vi "Recognize Starting Point.vi"() -> (0 "Sorted Waypoints":T1[](array[typedef]) {"Longitude" format="%#_14g"; "Latitude" format="%#_14g"}, 3 "Starting WP":T1={"Latitude"=2560.754484, "Longitude"=4991.702604} {"Longitude" format="%#_14g"; "Latitude" format="%#_14g"})   [LabVIEW 2009]
uses:
  TypeDefs/Sensor Typedefs/GPS Data.ctl
panel:
  out "Starting Point Index":i32=1
  out "Distances":dbl[](array[numeric])=[34.68592578168008, 0.0, 17.48374136365253]
  in  "NDIA GPS Pt":T1={"Latitude"=2560.745094, "Longitude"=4991.701278} {"Longitude" format="%#_14g"; "Latitude" format="%#_14g"}
  in  "SAIC GPS Pt":T1={"Latitude"=2560.754484, "Longitude"=4991.702604} {"Longitude" format="%#_14g"; "Latitude" format="%#_14g"}
  in  "Oakland GPS Pt":T1={"Latitude"=2560.7532, "Longitude"=4991.72802} {"Longitude" format="%#_14g"; "Latitude" format="%#_14g"}
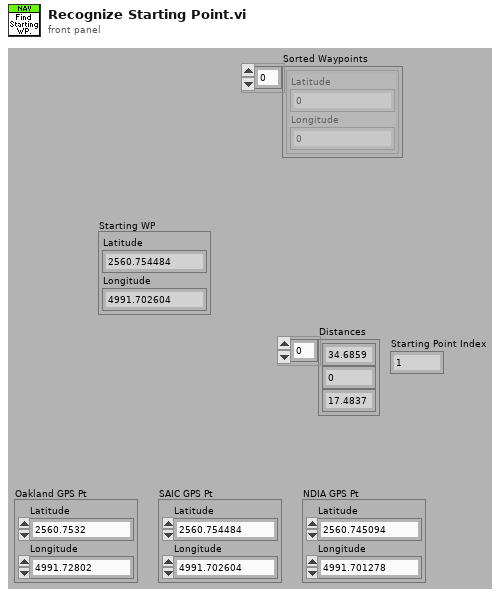
[diagram p1: front panel]
types:
  T1 = typedef "GPS Data.ctl" = cluster{"Latitude":dbl, "Longitude":dbl}
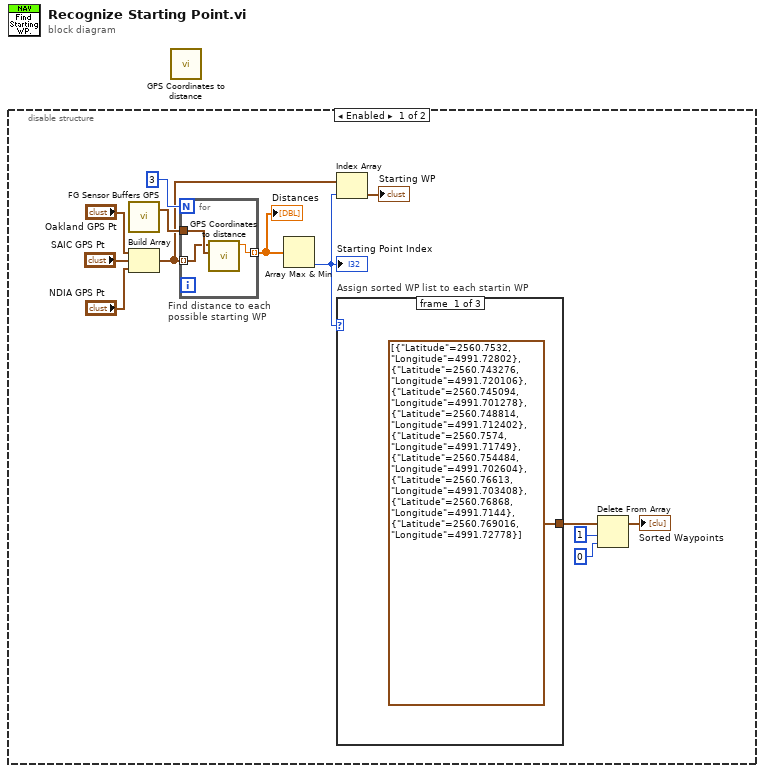
[diagram p0: block diagram]
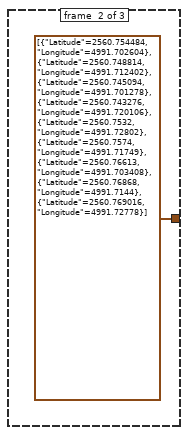
[diagram p2: hidden frame]
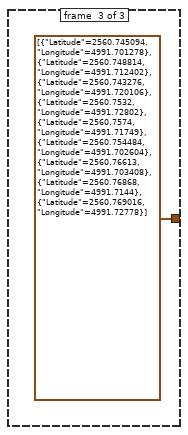
[diagram p3: hidden frame]
diagram:
  n1 = disable-structure shown="Enabled" {
    frame #0 {
      n2 = call "FG Sensor Buffers GPS.vi"() -> ("GPS Buffer out"=w13:T1)  [unwired: 3 in]
      n3 = Build Array("Oakland GPS Pt", "SAIC GPS Pt", "NDIA GPS Pt") -> (w7:T1[])
      n4 = for "Find distance to each\npossible starting WP" {
        N: 3 -> [_]
        tunnel: w13 -> [w19]
        tunnel: w7 -> [w18] mode=indexing
        tunnel: [w17] -> w8 mode=indexing
        n5 = call "GPS Coordinates to distance.vi"("GPS Co-ordinate 2"=w19, "GPS Co-ordinate 1"=w18) -> ("Distance"=w17:dbl)  [unwired: 9 in]
      }
      "Distances" <- w8
      n6 = Array Max & Min(array=w8) -> (min index (indices)=w5:i32)  [unwired: 3 out]
      "Starting Point Index" <- w5
      n7 = Index Array(array=w7, index=w5) -> (element=→"Starting WP":T1)
      n8 = case "Assign sorted WP list to each startin WP" shown="2" w5 {
        tunnel: [T1[] [{"Latitude"=2560.7532, "Longitude"=4991.72802}, {"Latitude"=2560.743276, "Longitude"=4991.720106}, {"Latitude"=2560.745094, "Longitude"=4991.701278}, {"Latitude"=2560.748814, "Longitude"=4991.712402}, {"Latitude"=2560.7574, "Longitude"=4991.71749}, {"Latitude"=2560.754484, "Longitude"=4991.702604}, {"Latitude"=2560.76613, "Longitude"=4991.703408}, {"Latitude"=2560.76868, "Longitude"=4991.7144}, {"Latitude"=2560.769016, "Longitude"=4991.72778}] T1[] [{"Latitude"=2560.754484, "Longitude"=4991.702604}, {"Latitude"=2560.748814, "Longitude"=4991.712402}, {"Latitude"=2560.745094, "Longitude"=4991.701278}, {"Latitude"=2560.743276, "Longitude"=4991.720106}, {"Latitude"=2560.7532, "Longitude"=4991.72802}, {"Latitude"=2560.7574, "Longitude"=4991.71749}, {"Latitude"=2560.76613, "Longitude"=4991.703408}, {"Latitude"=2560.76868, "Longitude"=4991.7144}, {"Latitude"=2560.769016, "Longitude"=4991.72778}] T1[] [{"Latitude"=2560.745094, "Longitude"=4991.701278}, {"Latitude"=2560.748814, "Longitude"=4991.712402}, {"Latitude"=2560.743276, "Longitude"=4991.720106}, {"Latitude"=2560.7532, "Longitude"=4991.72802}, {"Latitude"=2560.7574, "Longitude"=4991.71749}, {"Latitude"=2560.754484, "Longitude"=4991.702604}, {"Latitude"=2560.76613, "Longitude"=4991.703408}, {"Latitude"=2560.76868, "Longitude"=4991.7144}, {"Latitude"=2560.769016, "Longitude"=4991.72778}]] -> w4
        frame #0 {
        }
        frame #1 {
        }
        frame #2 {
        }
      }
      n9 = Delete From Array(array=w4, length=1, index=0) -> (array with subset deleted=→"Sorted Waypoints":T1[])  [unwired: 1 out]
    }
    frame #1 {
    }
  }
  n10 = call "GPS Coordinates to distance.vi"() -> ()  [unwired: 11 in, 1 out]
